vi "TCP (Writer).vi"(9 "data in":string, 10 "IP":string, 11 "Port":u16) -> (2 "error out":errorcluster, 3 "bytes written":i32)   [LabVIEW 2013]
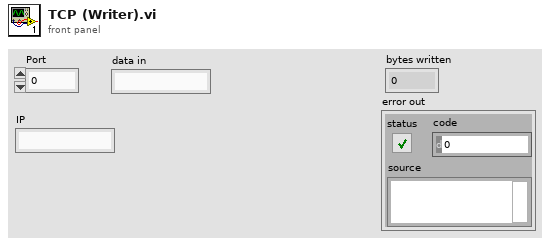
[diagram p1: front panel]
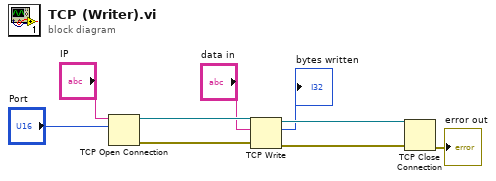
[diagram p0: block diagram]
diagram:
  n1 = TCP Open Connection(address="IP", remote port or service name="Port") -> (connection ID=w9:refnum<k5>, error out=w8:errorcluster)  [unwired: 3 in]
  n2 = TCP Write(connection ID=w9, data in="data in", error in (no error)=w8) -> (connection ID out=w7:refnum<k5>, bytes written=→"bytes written":i32, error out=w6:errorcluster)  [unwired: 1 in]
  n3 = TCP Close Connection(connection ID=w7, error in (no error)=w6) -> (error out=→"error out":errorcluster)  [unwired: 1 in, 1 out]
